vi "Call_enqueue.vi"(7 "Waveform":T6(array[cluster]), 8 "error in":errorcluster, 10 "Input Data":T1 {"Estimate Source" items=["Any Source."=-2, "No Shot"=-1, "Basic Labview Estimate"=0, "IDL Estimate From Andrew"=1, "IDL Estimate From Tobin"=2, "Old Metadata"=3]}, 11 "Timestamp":timestamp=timestamp(3428502400.8921742 s since 1904-01-01)) -> (0 "error out":errorcluster)   [LabVIEW 2013]
uses:
  User Interface/Controls/Hardware ID.ctl
  User Interface/Controls/Dust_Event.ctl
  User Interface/Controls/Signal.ctl
  User Interface/Controls/Role ID.ctl
  User Interface/Controls/Estimate_source.ctl
  <userlib>/_OpenG.lib/array/array.llb/Empty 1D Array (Variant)__ogtk.vi
panel:
  in  "First Detector\nHardware ID":T4=enum."CSA 2"
  in  "Second Detector\nHardware ID":T4=enum."CSA 3"
  in  "PSU Hardware ID":T4
  in  "Third Detector \nHardware ID":T4=enum."CSA 4"
  # "Dust Event"
  # "Signal"
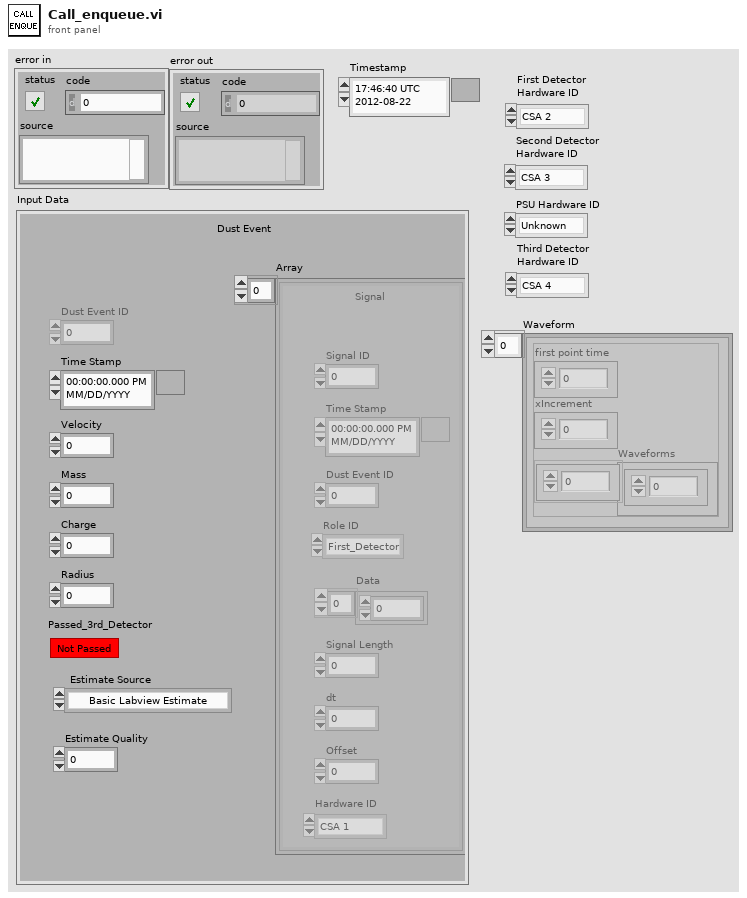
[diagram p1: front panel]
types:
  T1 = typedef "Dust_Event.ctl" = cluster{"Time Stamp":timestamp, "Velocity":sgl, "Mass":sgl, "Charge":sgl, "Radius":sgl, "Array":T2[], "Dust Event ID":i64, "Passed_3rd_Detector":bool, "Estimate Source":T5, "Estimate Quality":sgl}
  T2 = typedef "Signal.ctl" = cluster{"Signal ID":i64, "Time Stamp":timestamp, "Dust Event ID":i64, "Role ID":T3, "Data":sgl[], "Signal Length":i32, "dt":sgl, "Offset":dbl, "Hardware ID":T4}
  T3 = typedef "Role ID.ctl" = enum16{"First_Detector", "Second_Detector", "Third_Detector", "LeCroy_CH1", "LeCroy_CH2", "LeCroy_CH3", "LeCroy_CH4", "PSU", "DCS 1", "DCS 2"}
  T4 = typedef "Hardware ID.ctl" = enum16{"Unknown", "CSA 1", "CSA 2", "CSA 3", "CSA 4", "CSA 5", "CSA 6", "DCS 1", "DCS 2"}
  T5 = typedef "Estimate_source.ctl" = i8
  T6 = cluster{"first point time":dbl, "xIncrement":dbl, "Waveforms":dbl[]}[]
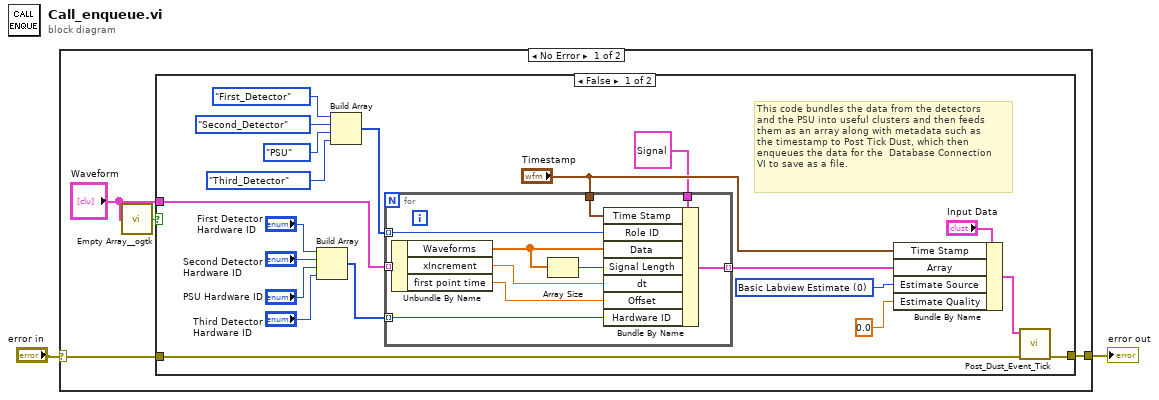
[diagram p0: block diagram]
diagram:
  n1 = case shown="No Error" "error in" {
    selector: "error in" -> [w5 w38]
    tunnel: [w6 w38] -> w1
    frame No Error {
      n2 = call-poly <userlib>:"Empty Array__ogtk.vi"("Array"="Waveform") -> ("Empty Array?"=w3:bool)  [unwired: 8 in]
      n3 = case shown="False" w3 {
        tunnel: "Waveform" -> [w18 _]
        tunnel: [w25 w37] -> w6
        tunnel: w5 -> [w19 w37]
        frame False {
          w24 = T5 0 items=["Basic Labview Estimate", "IDL Estimate"] ("Estimate Source")
          # "This code bundles the data from the detectors\nand the PSU into useful clusters and then feeds\nthem as an array along with metadata such as\nthe timestamp to Post Tick Dust, which then\nenqueues the data for the  Database Connection\nVI to save as a file."
          n4 = Build Array("First Detector\nHardware ID", "Second Detector\nHardware ID", "PSU Hardware ID", "Third Detector \nHardware ID") -> (w7:T4[])
          n5 = Build Array(Role_ID."First_Detector" ("Role ID"), Role_ID."Second_Detector" ("Role ID"), Role_ID."PSU" ("Role ID"), Role_ID."Third_Detector" ("Role ID")) -> (w8:T3[])
          n6 = for {
            tunnel: [w36] -> w17 mode=indexing
            tunnel: "Timestamp" -> [w35]
            tunnel: T2 {"Signal ID"=0, "Time Stamp"=timestamp(0 s since 1904-01-01), "Dust Event ID"=0, "Role ID"=enum."First_Detector", "Data"=[], "Signal Length"=0, "dt"=0.0, "Offset"=0.0, "Hardware ID"=enum."CSA 1"} ("Signal") -> [w34]
            tunnel: w18 -> [w29] mode=indexing
            tunnel: w8 -> [w28] mode=indexing
            tunnel: w7 -> [w27] mode=indexing
            n7 = Unbundle By Name(w29) -> ("Waveforms"=w32:dbl[], "xIncrement"=w30:dbl, "first point time"=w31:dbl)
            n8 = Array Size(array=w32) -> (size(s)=w33:i32)
            n9 = Bundle By Name(cluster=w34, "Time Stamp"=w35, "Role ID"=w28, "Data"=w32, "Signal Length"=w33, "dt"=w30, "Offset"=w31, "Hardware ID"=w27) -> (w36:T2)
          }
          n10 = Bundle By Name(cluster="Input Data", "Time Stamp"="Timestamp", "Array"=w17, "Estimate Source"=w24, "Estimate Quality"=sgl 0.0) -> (w26:T1)
          n11 = call "Post_Dust_Event_Tick.vi"("error in (no error)"=w19, "Input Data"=w26) -> ("error out"=w25:errorcluster)  [unwired: 8 in]
        }
        frame True {
        }
      }
    }
    frame Error {
    }
  }
  "error out" <- w1
